vi "Get Variable Name List.vi"(7 "Target (Process)":T1 items=["Process", "User", "Machine"], 8 "Error In":errorcluster) -> (0 "Error Out":errorcluster, 3 "Names[]":string[](array[string]))   [LabVIEW 2023, in "SLL Environment Variable.lvlib"]
doc: "Get the list of environment variables in the target environment."
uses:
  SLL Environment Variable.lvlib
  _Typedef/Target Environment Enum.ctl
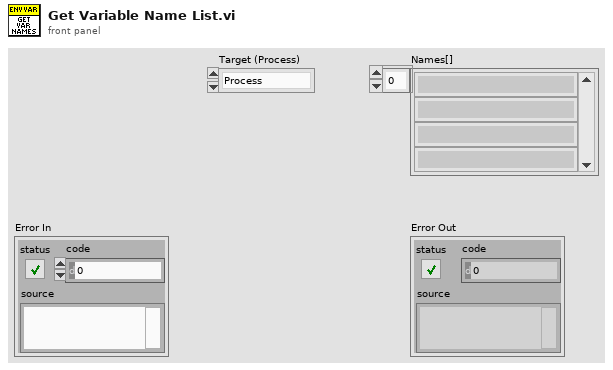
[diagram p1: front panel]
types:
  T1 = typedef "SLL Environment Variable.lvlib/Target Environment Enum.ctl" = i32
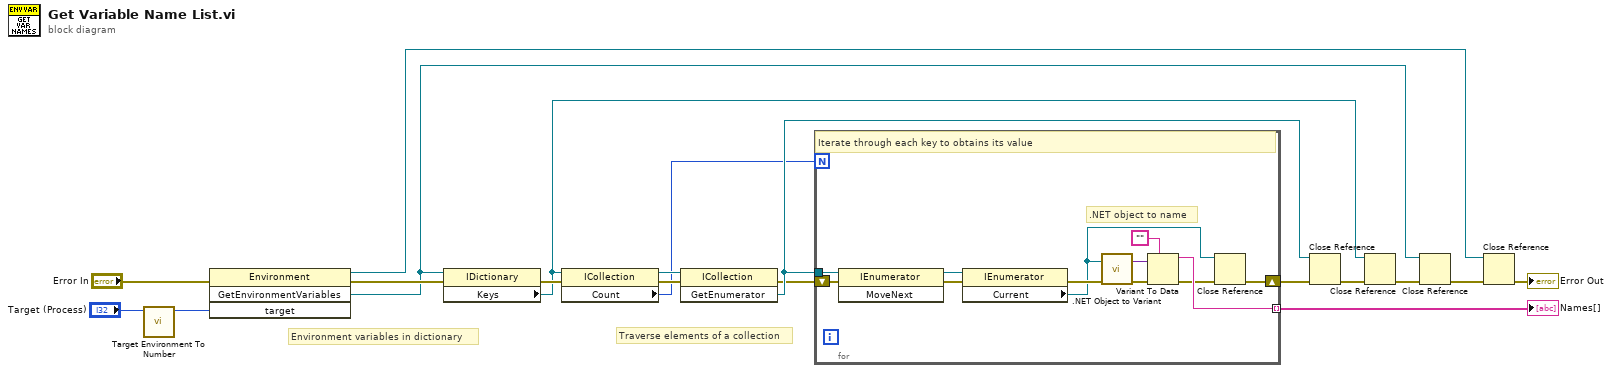
[diagram p0: block diagram]
diagram:
  # "Traverse elements of a collection"
  # "Environment variables in dictionary"
  n1 = call "Target Environment To Number.vi"("Target (Process)"="Target (Process)") -> ("Number"=w1:i32)  [unwired: 10 in]
  n2 = invoke class="Environment" method="GetEnvironmentVariables"(error in="Error In", "target"=w1) -> (reference out=w6:refnum<k24>, error out=w9:errorcluster, "GetEnvironmentVariables"=w8:refnum<k24>)  [unwired: 2 in, 1 out]
  n3 = property class="IDictionary"(reference=w8, error in=w9) -> (error out=w11:errorcluster, "Keys"=w5:refnum<k24>)  [unwired: 1 out]
  n4 = property class="ICollection"(reference=w5, error in=w11) -> (reference out=w13:refnum<k24>, error out=w12:errorcluster, "Count"=w4:i32)
  n5 = invoke class="ICollection" method="GetEnumerator"(reference=w13, error in=w12) -> (error out=w14:errorcluster, "GetEnumerator"=w15:refnum<k24>)  [unwired: 1 in, 1 out]
  n6 = for {
    N: w4 -> [_]
    tunnel: w15 -> [w27]
    tunnel: [w30] -> w3 mode=indexing
    shift-right: [w29] -> w19
    shift-left: w14 -> [w31]
    # ".NET object to name"
    # "Iterate through each key to obtains its value"
    n7 = invoke class="IEnumerator" method="MoveNext"(reference=w27, error in=w31) -> (reference out=w20:refnum<k24>, error out=w28:errorcluster)  [unwired: 1 in, 1 out]
    n8 = property class="IEnumerator"(reference=w20, error in=w28) -> (error out=w26:errorcluster, "Current"=w21:refnum<k24>)  [unwired: 1 out]
    n9 = call <vilib>:".NET Object to Variant.vi"("error in (no error)"=w26, ".NET object"=w21) -> ("error out"=w25:errorcluster, "variant"=w24:variant)
    n10 = Variant To Data(error in=w25, type="", Variant=w24) -> (data=w30:string, error out=w23:errorcluster)
    n11 = Close Reference(reference=w21, error in (no error)=w23) -> (error out=w29:errorcluster)
  }
  "Names[]" <- w3
  n12 = Close Reference(reference=w15, error in (no error)=w19) -> (error out=w16:errorcluster)
  n13 = Close Reference(reference=w5, error in (no error)=w16) -> (error out=w17:errorcluster)
  n14 = Close Reference(reference=w8, error in (no error)=w17) -> (error out=w18:errorcluster)
  n15 = Close Reference(reference=w6, error in (no error)=w18) -> (error out=→"Error Out":errorcluster)
